vi "Add AI.vi"(8 "error in (no error)":errorcluster, 10 "Physical Channel Number":i32, 11 "Device Item Ref in":T1 format="%.0x") -> (0 "error out":errorcluster, 3 "Parent Ref out":T1 format="%.0x")   [LabVIEW 2020, in "NI PXIe-4340 System Explorer.lvlib"]
doc: "Add an Analog Output channel based on the physical channel specified"
uses:
  NI PXIe-4340 System Explorer.lvlib
  <vilib>/NI VeriStand/Custom Device API/Custom Device Item Ref.ctl
  <vilib>/NI VeriStand/Custom Device API/Custom Device Channel.ctl
  <vilib>/NI VeriStand/Custom Device API/Custom Device Channel Type.ctl
  Shared/Constants.vi
  <vilib>/NI VeriStand/Custom Device API/Custom Device API.lvlib
  Shared/NI PXIe-4340 Shared.lvlib
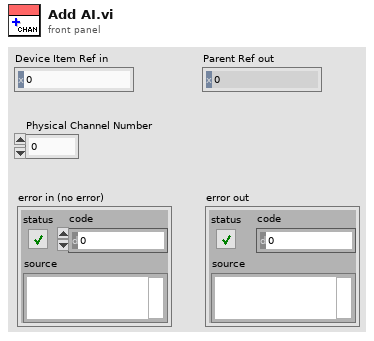
[diagram p1: front panel]
types:
  T1 = typedef "Custom Device API.lvlib/Custom Device Item Ref.ctl" = u64
  T2 = typedef "Custom Device API.lvlib/Custom Device Channel.ctl" = cluster{"Type":T3, "Units":string, "Default Value":dbl, "Faultable":bool, "Scalable":bool}
  T3 = typedef "Custom Device API.lvlib/Custom Device Channel Type.ctl" = enum16{"Input", "Output"}
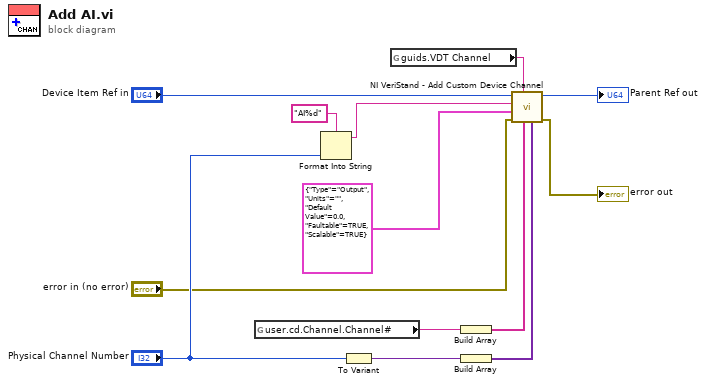
[diagram p0: block diagram]
diagram:
  n1 = global read "Constants.vi" "user.cd.Channel.Channel#"() -> (w10:string)
  n2 = Format Into String(format string="AI%d", "Physical Channel Number") -> (resulting string=w3:string)  [unwired: 2 in, 1 out]
  n3 = To Variant(anything="Physical Channel Number") -> (Variant=w12:variant)
  n4 = global read "Constants.vi" "guids.VDT Channel"() -> (w4:string)
  n5 = Build Array(w10) -> (w2:string[])
  n6 = Build Array(w12) -> (w1:variant[])
  n7 = call <vilib>:"NI VeriStand - Add Custom Device Channel.vi"("Property Values"=w1, "Property names"=w2, "GUID (Default Channel)"=w4, "error in (no error)"="error in (no error)", "Channel"=T2 {"Type"=enum."Output", "Units"="", "Default Value"=0.0, "Faultable"=TRUE, "Scalable"=TRUE}, "Channel Name"=w3, "Parent Ref in"="Device Item Ref in") -> ("error out"=→"error out":errorcluster, "Parent Ref out"=→"Parent Ref out":T1)  [unwired: 1 in, 2 out]
